vi "AMX-电源头正面标签漏线检测参数读取.vi"(7 "error in (no error)":errorcluster caption="错误输入（无错误）", 10 "基路径":path) -> (0 "error out":errorcluster caption="错误输出", 2 "颗粒物检测1参数":T2={"Rectangle"={"Left"=0, "Top"=0, "Right"=0, "Bottom"=0, "Rotation"=0.0}, "模板路径"=path "C:/Users/delluser001/Desktop/PowerLine Inspect System/Source Code/Template Program/potteryTemplete/Color.png", "Match Mode "=0, "Minimum Match Score "=800.0, "Number of Matches Requested"=1, "Rotation Angle Ranges (degrees)"=[{"Min"=-180.0, "Max"=180.0}], "Color Sensitivity "=0, "Match Offset"={"X"=0.0, "Y"=0.0}, "Color Score Weight "=500.0, "Search Strategy "=0, "Subpixel Accuracy "=FALSE} {"Rectangle"."Rotation" format="%.2f"; "Rectangle"."Left" scale=0.0..1024.0; "Rectangle"."Right" scale=0.0..1024.0; "Search Strategy" items=["Conservative", "Balance", "Aggressive", "Very Aggressive"]; "Color Sensitivity" items=["Low Sensitivity", "Medium Sensitivity", "High Sensitivity"]; "Match Mode" items=["Shift Invariant", "Rotation Invariant"]}, 3 "颗粒物检测1基础参数":T3={"IsNorImage"=TRUE, "Exposure Values"=100289, "ImagePath"=path "C:/Users/hedongpo/Desktop/514-hdp/Alignment Assemble System/Test Picture/B/3.bmp"} caption="参数界面" {"Exposure Values" scale=0.0..200000.0})   [LabVIEW 2017]
uses:
  <vilib>/Utility/xml.llb/Read From XML File(string).vi
  Global System.vi
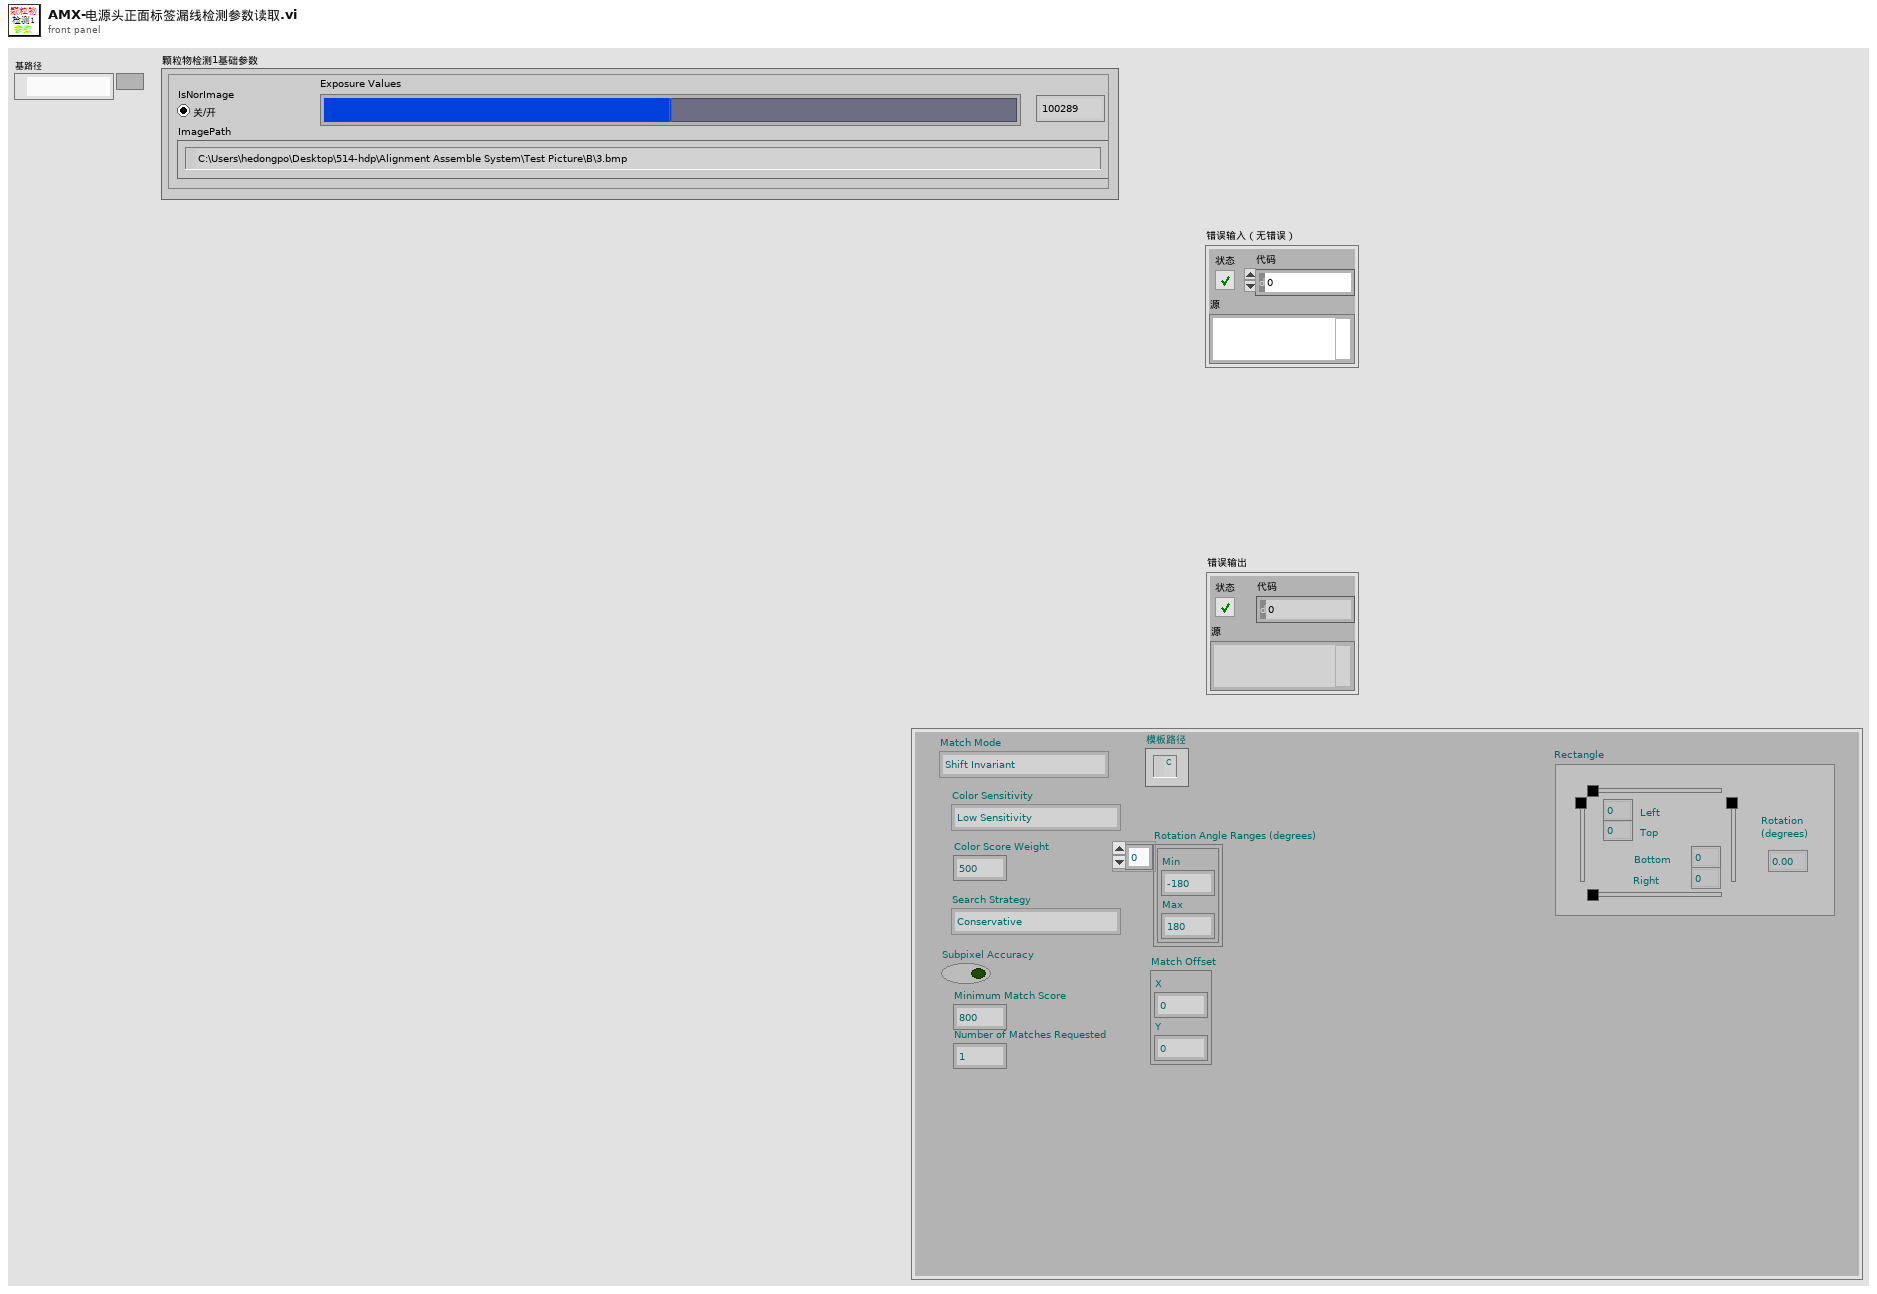
[diagram p1: front panel]
types:
  T1 = typedef "IMAQ Rectangle" = cluster{"Left":i32, "Top":i32, "Right":i32, "Bottom":i32, "Rotation":dbl}
  T2 = cluster{"Rectangle":T1, "模板路径":path, "Match Mode ":u32, "Minimum Match Score ":sgl, "Number of Matches Requested":i32, "Rotation Angle Ranges (degrees)":cluster{"Min":sgl, "Max":sgl}[], "Color Sensitivity ":u32, "Match Offset":cluster{"X":sgl, "Y":sgl}, "Color Score Weight ":sgl, "Search Strategy ":u32, "Subpixel Accuracy ":bool}
  T3 = cluster{"IsNorImage":bool, "Exposure Values":u32, "ImagePath":path}
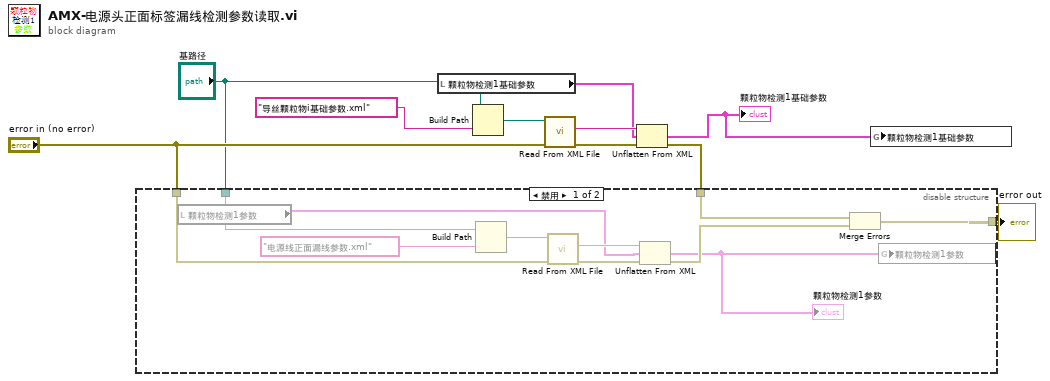
[diagram p0: block diagram]
diagram:
  n1 = local read "颗粒物检测1基础参数"() -> (w3:T3)
  n2 = Build Path(base path="基路径", name or relative path="导丝颗粒物i基础参数.xml" ("名称或相对路径")) -> (appended path=w10:path)
  n3 = call-poly <vilib>:"Read From XML File.vi"("error in (no error)"="error in (no error)", "XML File Path"=w10) -> ("error out"=w7:errorcluster, "XML Elements"=w9:string)  [unwired: 7 in, 1 out]
  n4 = Unflatten From XML(xml string=w9, type=w3, error in (no error)=w7) -> (value=w1:T3, error out=w6:errorcluster)
  "颗粒物检测1基础参数" <- w1
  n5 = disable-structure shown="禁用" {
    disable-tunnel: "error in (no error)" -> [w19 _]
    disable-tunnel: w6 -> [w18 _]
    disable-tunnel: [w15 _] -> w5
    disable-tunnel: "基路径" -> [w14 _]
    frame Disabled {
      n6 = local read "颗粒物检测1参数"() -> (w12:T2)
      n7 = Build Path(base path=w14, name or relative path="电源线正面漏线参数.xml" ("名称或相对路径")) -> (appended path=w20:path)
      n8 = call-poly <vilib>:"Read From XML File.vi"("error in (no error)"=w19, "XML File Path"=w20) -> ("error out"=w17:errorcluster, "XML Elements"=w21:string)  [unwired: 7 in, 1 out]
      n9 = Unflatten From XML(xml string=w21, type=w12, error in (no error)=w17) -> (value=w11:T2, error out=w16:errorcluster)
      "颗粒物检测1参数" <- w11
      n10 = Merge Errors(w18, w16) -> (w15:errorcluster)
      n11 = global write "Global System.vi" "颗粒物检测1参数"(w11) -> ()
    }
    frame Enabled {
    }
  }
  "error out" <- w5
  n12 = global write "Global System.vi" "颗粒物检测1基础参数"(w1) -> ()
